vi "Find All SLSC Switch Custom Devices.vi"(8 "error in":errorcluster, 11 "slsc chassis in":T1 format="%.0x") -> (0 "error out":errorcluster, 2 "slsc switch custom devices":T1[](array[typedef]) format="%.0x", 3 "slsc chassis out":T1 format="%.0x")   [LabVIEW 2019, in "SLSC Switch Scripting.lvlib"]
doc: "Returns all SLSC Switch custom devices under the SLSC chassis."
uses:
  SLSC Switch Scripting.lvlib
  <vilib>/NI VeriStand/Custom Device API/Custom Device Item Ref.ctl
  Shared/Constants.vi
  Shared/SLSC Switch Shared.lvlib
  Shared/VeriStand SLSC Scripting/VeriStand SLSC Scripting.lvlib
  <vilib>/NI VeriStand/Custom Device API/Custom Device API.lvlib
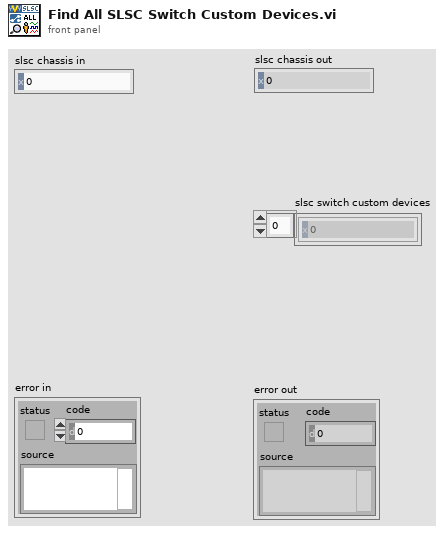
[diagram p1: front panel]
types:
  T1 = typedef "Custom Device API.lvlib/Custom Device Item Ref.ctl" = u64
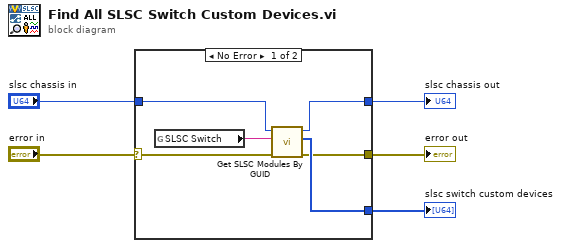
[diagram p0: block diagram]
diagram:
  n1 = case shown="No Error" "error in" {
    selector: "error in" -> [w11 w13]
    tunnel: [w9 w13] -> w4
    tunnel: [w10 _] -> w3
    tunnel: "slsc chassis in" -> [w6 w12]
    tunnel: [w7 w12] -> w1
    frame No Error {
      n2 = global read "Constants.vi" "SLSC Switch"() -> (w8:string)
      n3 = call "Get SLSC Modules By GUID.vi"("error in (no error)"=w11, "GUID"=w8, "SLSC Chassis"=w6) -> ("error out"=w9:errorcluster, "SLSC Modules"=w10:u64[], "SLSC Chassis out"=w7:u64)  [unwired: 5 in, 1 out]
    }
    frame Error {
    }
  }
  "error out" <- w4
  "slsc switch custom devices" <- w3
  "slsc chassis out" <- w1
